vi "read_y.vi"(8 "error in (no error)":errorcluster, 11 "OrthogonalMatchingPursuit in":refnum<class "OrthogonalMatchingPursuit.lvclass">) -> (0 "error out":errorcluster, 2 "y":dbl[][](array[numeric]), 3 "OrthogonalMatchingPursuit out":refnum<class "OrthogonalMatchingPursuit.lvclass">)   [LabVIEW 2020, in "OrthogonalMatchingPursuit.lvclass"]
uses:
  OrthogonalMatchingPursuit.lvclass
  OrthogonalMatchingPursuit.lvclass/OrthogonalMatchingPursuit.ctl
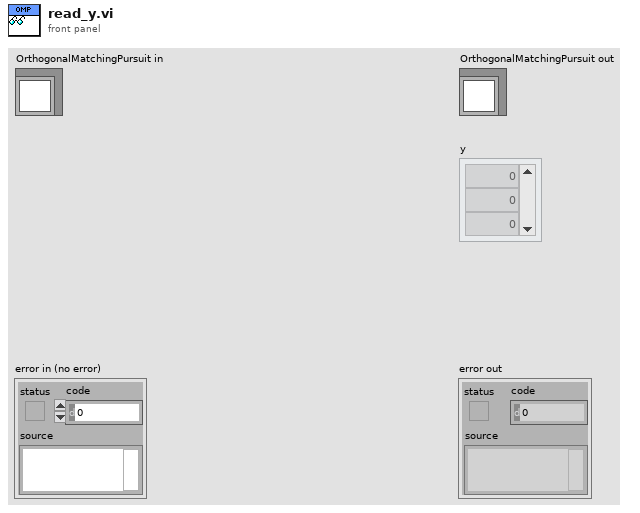
[diagram p1: front panel]
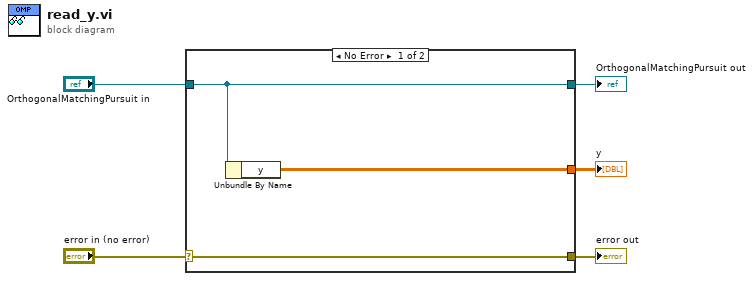
[diagram p0: block diagram]
diagram:
  n1 = case shown="No Error" "error in (no error)" {
    selector: "error in (no error)" -> [w8 w9]
    tunnel: [w8 w9] -> w4
    tunnel: [w7 w10] -> w2
    tunnel: "OrthogonalMatchingPursuit in" -> [w7 w10]
    tunnel: [w6 _] -> w1
    frame No Error {
      n2 = Unbundle By Name(w7) -> ("y"=w6:dbl[][])
    }
    frame Error {
    }
  }
  "error out" <- w4
  "OrthogonalMatchingPursuit out" <- w2
  "y" <- w1
